vi "ChangeColorByTime.vi"(9 "Target Color":u32(colorbox)=9502720, 10 "Base Color":u32(colorbox)=2829099, 11 "ms":u32) -> (2 "Result Color":u32(colorbox)=2829099)   [LabVIEW 2015]
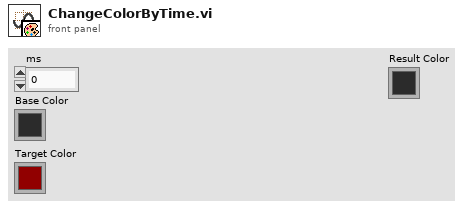
[diagram p1: front panel]
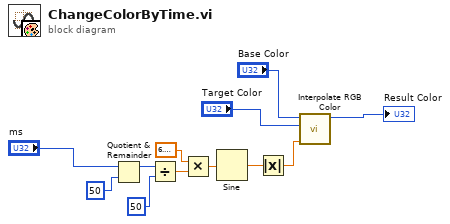
[diagram p0: block diagram]
diagram:
  n1 = Quotient & Remainder(x="ms", y=u32 50 ("milliseconds to wait")) -> (x-y*floor(x/y)=w9:u32)  [unwired: 1 out]
  n2 = Divide(x=w9, y=u32 50 ("milliseconds to wait")) -> (x/y=w6:dbl)
  n3 = Multiply(x=6.283185307179586, y=w6) -> (x*y=w11:dbl)
  n4 = Sine(x=w11) -> (sin(x)=w10:dbl)
  n5 = Absolute Value(x=w10) -> (abs(x)=w5:dbl)
  n6 = call "Interpolate RGB Color.vi"("Proportion"=w5, "Target Color"="Target Color", "Base Color"="Base Color") -> ("Result Color"=→"Result Color":u32)  [unwired: 8 in]
